vi "Untitled 2.vi"() -> ()   [LabVIEW 2013]
panel:
  out "Waveform Chart 2":i16(graph)
  out "Waveform Chart":i16(graph)
  out "Счетчик частоты":i32
  out "Счетчик данных":i16
  out "CLK":bool
  out "DATA":bool
  out "WE":bool
  out "ACK":bool[](array[boolean])
  in  "DataLow":u64
  in  "DataUp":u64
  in  "100_Sclk_divider":i32=25
  out "Sclk":bool
  in  "75_Stop":i16=57
  in  "53":i16=53
  in  "35":i16=35
  in  "17":i16=17
  in  "71":i16=53
  in  "54":i16=53
  in  "36":i16=35
  in  "18":i16=17
  in  "72":i16=53
  in  "10_Rise/Fall divider":i32=3
  in  "0_WE divider":i32=10
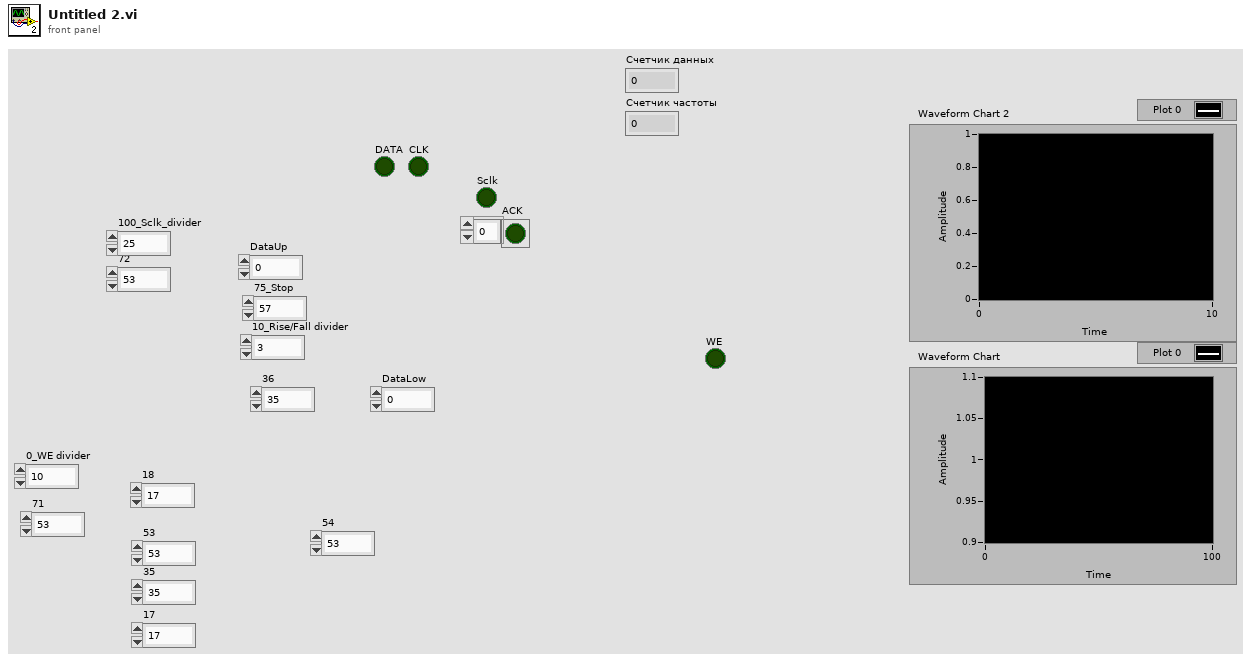
[diagram p1: front panel]
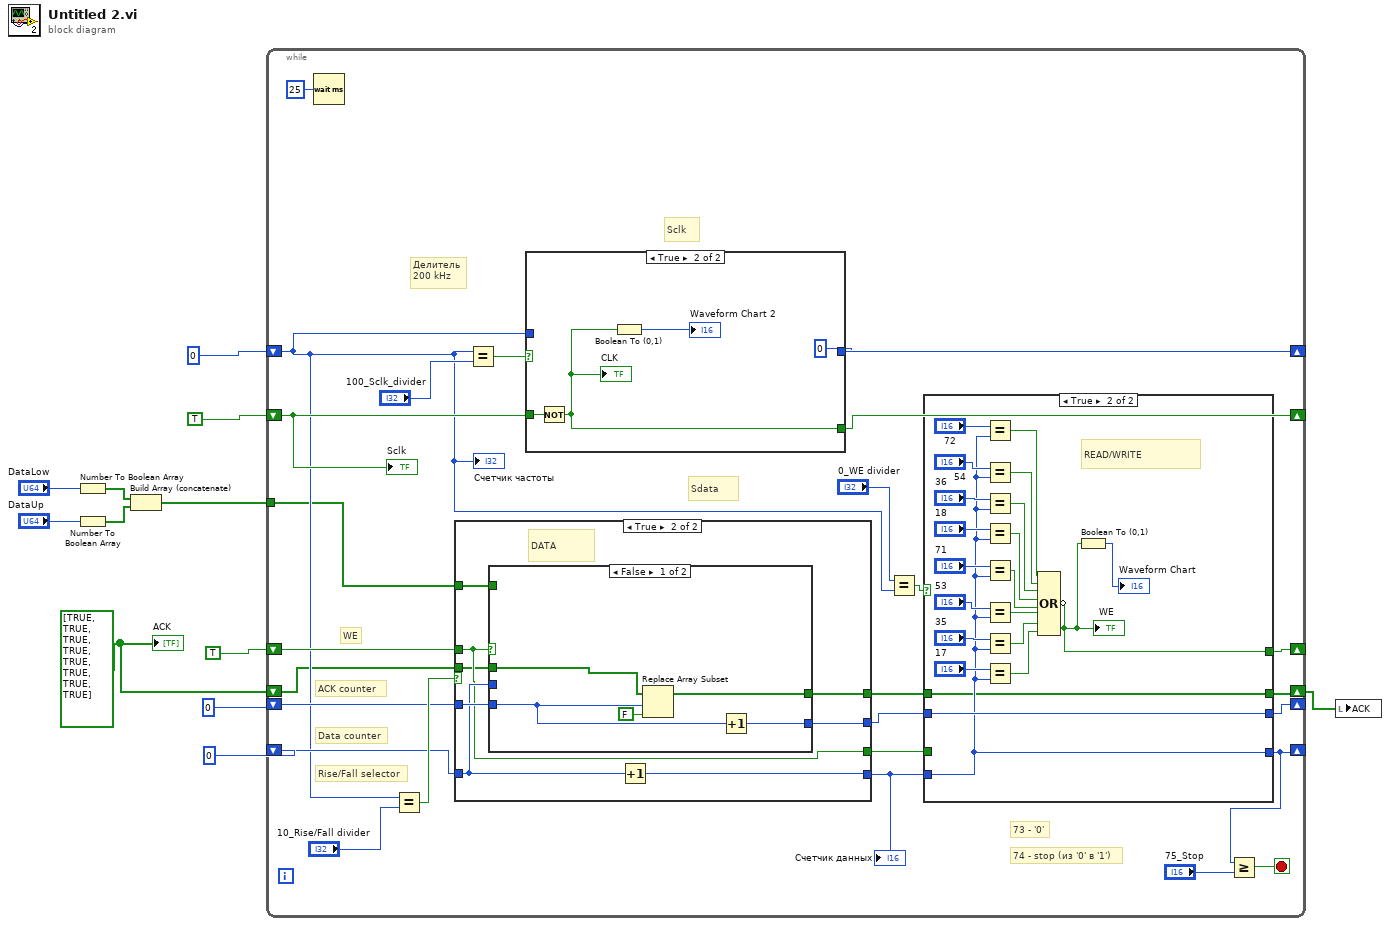
[diagram p0: block diagram]
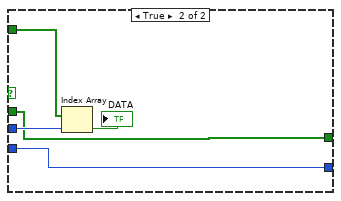
[diagram p4: hidden frame]
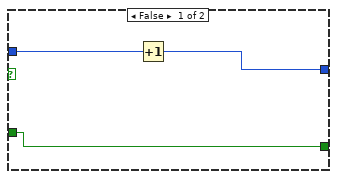
[diagram p5: hidden frame]
diagram:
  w2 = bool[] [TRUE, TRUE, TRUE, TRUE, TRUE, TRUE, TRUE, TRUE] ("ACK")
  n1 = Number To Boolean Array(number="DataLow") -> (Boolean array=w8:bool[])
  n2 = Number To Boolean Array(number="DataUp") -> (Boolean array=w7:bool[])
  n3 = Build Array (concatenate)(w8, w7) -> (w1:bool[])
  n4 = while {
    shift-right: [w37] -> _
    shift-left: 0 -> [w26]
    shift-right: [w36] -> _
    shift-left: TRUE ("IO Module\\DDCA_DIO0_Write") -> [w33]
    shift-right: [w23] -> _
    shift-left: i16 0 -> [w31]
    shift-right: [w21] -> _
    shift-left: i16 0 -> [w30]
    shift-right: [w20] -> _
    shift-left: TRUE -> [w29]
    shift-right: [w16] -> w3
    shift-left: w2 -> [w15]
    tunnel: w1 -> [w13]
    stop <- w18 stop-if-true
    # "Rise/Fall selector"
    # "WE"
    # "Data counter"
    # "ACK counter"
    # "74 - stop (из '0' в '1')"
    # "73 - '0'"
    # "Sdata"
    # "Sclk"
    # "Делитель\n200 kHz"
    n5 = Wait (ms)(milliseconds to wait=u32 25) -> ()  [unwired: 1 out]
    n6 = Equal?(x=w26, y="10_Rise/Fall divider") -> (x = y?=w32:bool)
    n7 = case shown="True" w32 {
      tunnel: [w66 w71] -> w24
      tunnel: w31 -> [w66 w73]
      tunnel: w30 -> [w67 w75]
      tunnel: [w67 w74] -> w22
      tunnel: w29 -> [w65 w72]
      tunnel: [w65 w72] -> w19
      tunnel: [w64 w70] -> w17
      tunnel: w15 -> [w64 w69]
      tunnel: w13 -> [_ w68]
      frame False {
      }
      frame True {
        # "DATA"
        n8 = case shown="False" w72 {
          tunnel: w75 -> [w80 w85]
          tunnel: [w79 w85] -> w74
          tunnel: w73 -> [_ w84]
          tunnel: [w78 w83] -> w70
          tunnel: w69 -> [w77 w83]
          tunnel: w68 -> [_ w82]
          frame False {
            n9 = Replace Array Subset(array=w77, new element=FALSE ("new element/subarray"), index=w80) -> (w78:bool[])
            n10 = Increment(x=w80) -> (x+1=w79:i16)
          }
          frame True {
            n11 = Index Array(array=w82, index=w84) -> (element=→"DATA":bool)
          }
        }
        n12 = Increment(x=w73) -> (x+1=w71:i16)
      }
    }
    "Счетчик данных" <- w24
    n13 = Equal?(x=w26, y="100_Sclk_divider") -> (x = y?=w38:bool)
    n14 = case shown="True" w38 {
      tunnel: [w87 0] -> w37
      tunnel: w26 -> [w88 _]
      tunnel: w33 -> [w86 w91]
      tunnel: [w86 w89] -> w36
      frame False {
        n15 = Increment(x=w88) -> (x+1=w87:i32)
      }
      frame True {
        n16 = Not(x=w91) -> (.not. x?=w89:bool)
        "CLK" <- w89
        n17 = Boolean To (0,1)(Boolean=w89) -> (0, 1=→"Waveform Chart 2":i16)
      }
    }
    n18 = Equal?(x="0_WE divider", y=w26) -> (x = y?=w25:bool)
    n19 = case shown="True" w25 {
      tunnel: w24 -> [w41 w50]
      tunnel: [w41 w50] -> w23
      tunnel: [w42 w55] -> w21
      tunnel: w22 -> [w42 w55]
      tunnel: [w40 w44] -> w20
      tunnel: w19 -> [w40 _]
      tunnel: w17 -> [w39 w45]
      tunnel: [w39 w45] -> w16
      frame False {
      }
      frame True {
        # "READ/WRITE"
        n20 = Equal?(x="72", y=w50) -> (x = y?=w49:bool)
        n21 = Equal?(x="54", y=w50) -> (x = y?=w46:bool)
        n22 = Equal?(x="36", y=w50) -> (x = y?=w48:bool)
        n23 = Equal?(x="18", y=w50) -> (x = y?=w47:bool)
        n24 = Equal?(x="71", y=w50) -> (x = y?=w56:bool)
        n25 = Equal?(x="53", y=w50) -> (x = y?=w59:bool)
        n26 = Equal?(x="35", y=w50) -> (x = y?=w61:bool)
        n27 = Equal?(x="17", y=w50) -> (x = y?=w63:bool)
        n28 = Compound Arithmetic op=OR(w49, w46, w48, w47, w56, w59, w61, w63) -> (invert w44:bool)
        "WE" <- w44
        n29 = Boolean To (0,1)(Boolean=w44) -> (0, 1=→"Waveform Chart":i16)
      }
    }
    n30 = Greater Or Equal?(x=w23, y="75_Stop") -> (x >= y?=w18:bool)
    "Sclk" <- w33
    "Счетчик частоты" <- w26
  }
  n31 = local write "ACK"(w3) -> ()
  "ACK" <- w2
